vi "C843_Sample_Application_1_RE.vi"() -> ()   [LabVIEW 2011]
doc: "This VI demonstrates how to statically define a C-843 configuration with connected axes. In this example an M-405.PD stage is attached to axis 1, an M-126.PD to axis 2 and an M-037.PD to axis 3. The VI runs C843_Configuration_Setup.vi with these specified settings and reads the position of all axes. The diagram shows how to combine the driver VIs for these tasks. \nWarning: Before running this VI, modify the \"Stage names input\" array to reflect your configuration. The predefined settings provided with the VI probably do not match your system."
panel:
  in  "stop":bool
  in  "error in":errorcluster
  out "Running":bool caption="Axes are referencing"
  out "error out":errorcluster
  out "Position":dbl[](array[numeric]) format="%.6f"
  out "Conn. Axes":string[](array[string])
  out "Identification":string
  # "Simple C-843 sample program"
  # "This VI demonstrates how to statically define a C-843 configuration with connected axes. In this example an M-405.PD stage is attached\nto axis 1, an M-126.PD to axis 2 and an M-037.PD to axis 3. The VI runs C843_Configuration_Setup.vi with these specified settings and reads the position \nof all axes. The diagram shows how to combine the driver VIs for these tasks. \n\nWarning: Before running this VI, modify the \"Stage names input\" array to reflect your configuration. The predefined settings provided \n                 with the VI probably do not match your system."
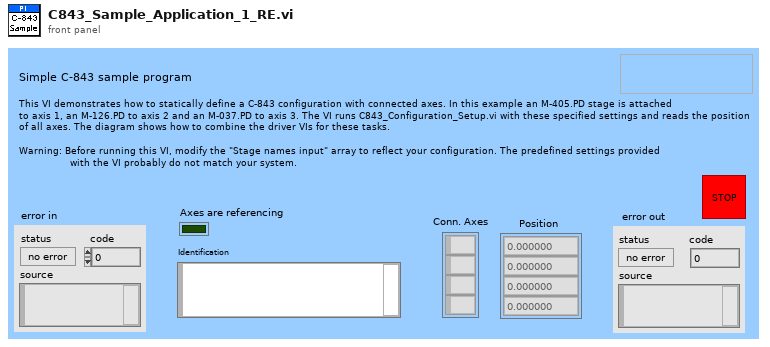
[diagram p1: front panel]
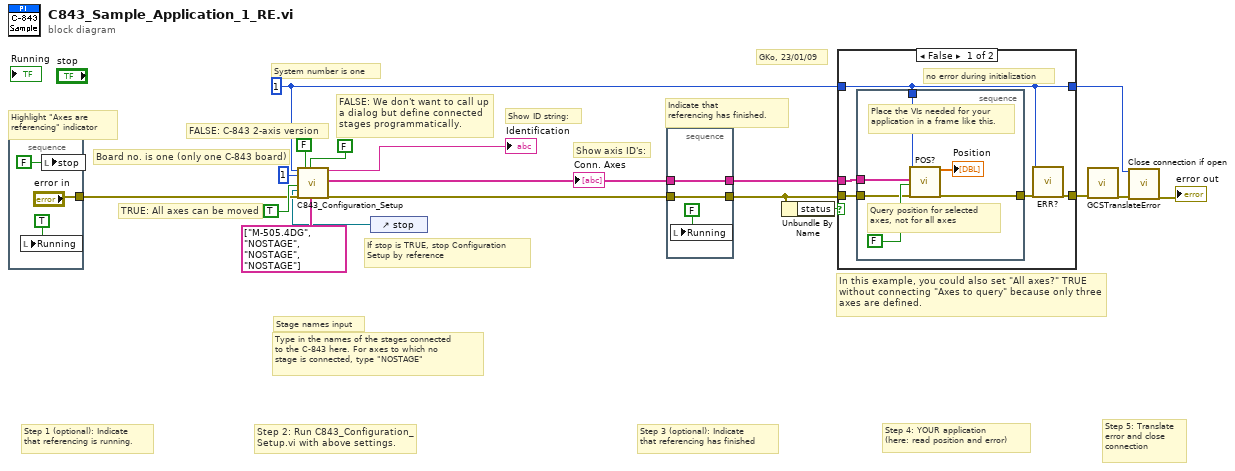
[diagram p0: block diagram]
diagram:
  w8 = 1 ("System no.")
  # "Step 5: Translate\nerror and close\nconnection"
  # "In this example, you could also set \"All axes?\" TRUE \nwithout connecting \"Axes to query\" because only three\naxes are defined."
  # "If stop is TRUE, stop Configuration\nSetup by reference"
  # "Type in the names of the stages connected\nto the C-843 here. For axes to which no \nstage is connected, type \"NOSTAGE\""
  # "Stage names input"
  # "GKo, 23/01/09"
  # "Step 4: YOUR application\n(here: read position and error)"
  # "Step 3 (optional): Indicate\nthat referencing has finished"
  # "Step 2: Run C843_Configuration_\nSetup.vi with above settings."
  # "Step 1 (optional): Indicate\nthat referencing is running."
  # "Indicate that\nreferencing has finished."
  # "Highlight \"Axes are\nreferencing\" indicator"
  # "Show axis ID's:"
  # "Show ID string:"
  # "FALSE: We don't want to call up\na dialog but define connected \nstages programmatically."
  # "TRUE: All axes can be moved"
  # "Board no. is one (only one C-843 board)"
  # "System number is one"
  # "FALSE: C-843 2-axis version"
  n1 = stacked-sequence {
    tunnel: ["error in"] -> w10
    frame #0 {
      n2 = local write "Running"(TRUE ("Running")) -> ()
      n3 = local write "stop"(FALSE ("stop")) -> ()
    }
  }
  n4 = control-ref of="stop"() -> (w9:refnum<vi>)
  n5 = call "C843_Configuration_Setup.vi"("System no."=w8, "C-843 Board No."=1, "All axes?"=TRUE, "Stop refnum"=w9, "error in"=w10, "C-843 version"=FALSE, "Use dialog to define\nconnected stages?"=FALSE ("Use dialog to define\nconnected stages?"), "Stage names input"=string[] ["M-505.4DG", "NOSTAGE", "NOSTAGE", "NOSTAGE"]) -> ("Identification"=→"Identification":string, "Conn. \nAxes"=w12:string[], "error out"=w11:errorcluster)  [unwired: 7 in, 2 out]
  "Conn. Axes" <- w12
  n6 = stacked-sequence {
    tunnel: w12 -> [w24]
    tunnel: [w24] -> w5
    tunnel: w11 -> [w23]
    tunnel: [w23] -> w6
    frame #0 {
      n7 = local write "Running"(FALSE ("Running")) -> ()
    }
  }
  n8 = Unbundle By Name(w6) -> ("status"=w7:bool)
  n9 = case shown="False" w7 {
    tunnel: [w25 w37] -> w2
    tunnel: w6 -> [w29 w37]
    tunnel: w8 -> [w26 w36]
    tunnel: w5 -> [w27 _]
    tunnel: [w26 w36] -> w3
    frame False {
      # "no error during initialization"
      n10 = stacked-sequence {
        tunnel: w26 -> [w35]
        tunnel: w29 -> [w33]
        tunnel: [w32] -> w28
        tunnel: w27 -> [w30]
        frame #0 {
          # "Place the VIs needed for your\napplication in a frame like this."
          # "Query position for selected\naxes, not for all axes"
          n11 = call "POS?.vi"("System no."=w35, "Axes to query"=w30, "All axes?"=FALSE, "error in"=w33) -> ("Position"=→"Position":dbl[], "error out"=w32:errorcluster)  [unwired: 14 in]
        }
      }
      n12 = call "ERR?.vi"("System no."=w26, "error in"=w28) -> ("error out"=w25:errorcluster)  [unwired: 16 in, 1 out]
    }
    frame True {
      # "Error during initialization,\nstop execution here."
    }
  }
  n13 = call "GCSTranslateError.vi"("error in"=w2) -> ("error out"=w1:errorcluster)  [unwired: 16 in, 2 out]
  n14 = call "Close connection if open.vi"("System no."=w3, "error in"=w1) -> ("error out"=→"error out":errorcluster)  [unwired: 16 in, 1 out]
